vi "Record Measurement.vi"(0 "Linear Density":dbl, 1 "Operator ID":i32, 2 "sMDT Code":string, 4 "Wire Length":dbl, 6 "Tension":dbl, 7 "User List":string[](array[string]), 8 "Uncertainty":dbl, 9 "Frequency":dbl, 10 "Nth measurement":i32, 11 "t < X ?":bool) -> (3 "Measurements":string[][](array[string]))   [LabVIEW 2018]
panel:
  # "Inputs"
  # "Outputs"
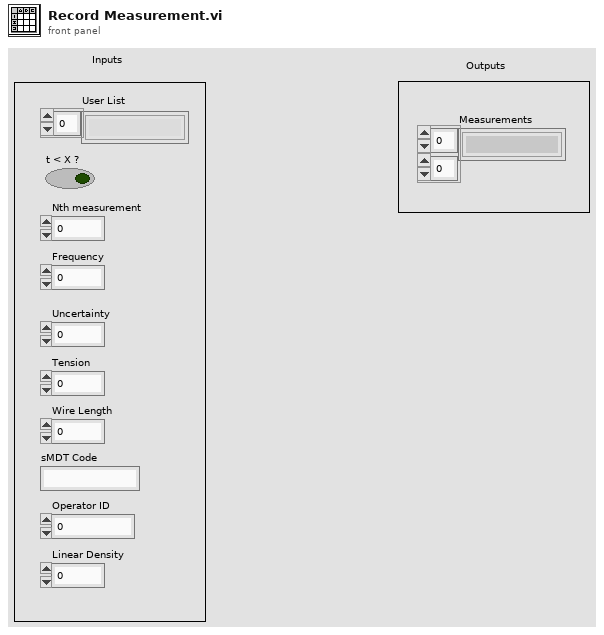
[diagram p1: front panel]
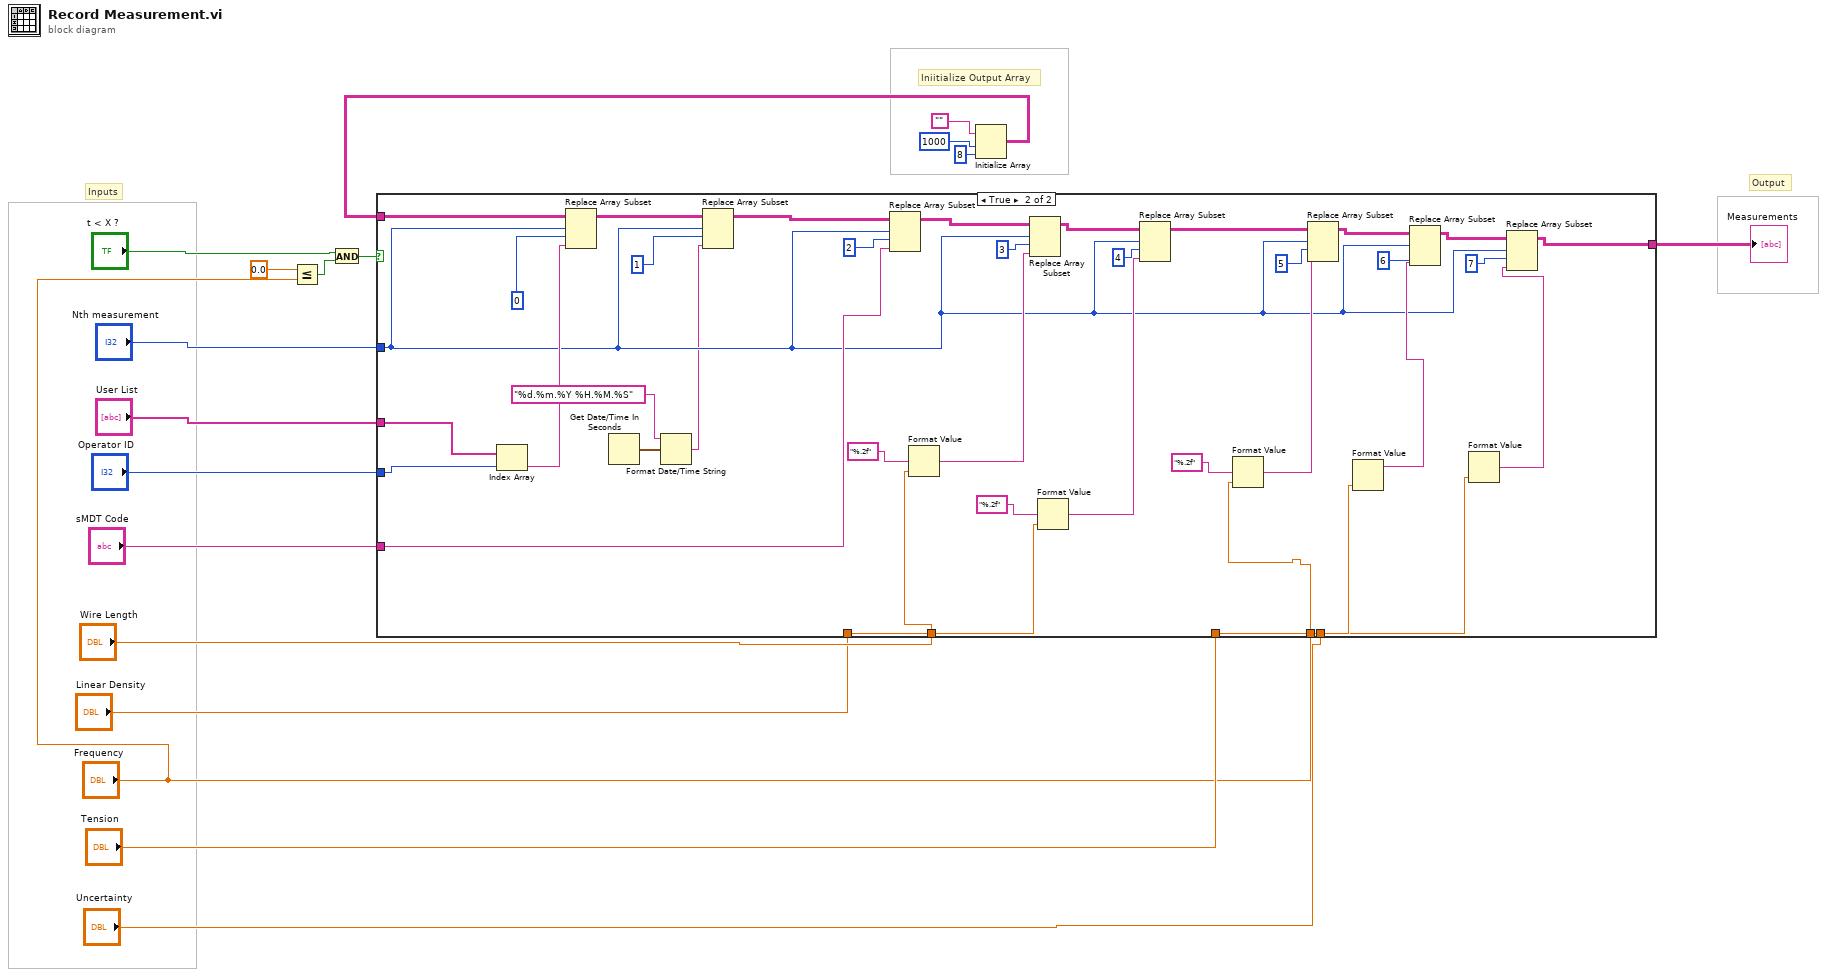
[diagram p0: block diagram]
diagram:
  # "Output"
  # "Inputs"
  # "Iniitialize Output Array"
  n1 = Less Or Equal?(x=0.0, y="Frequency") -> (x <= y?=w5:bool)
  n2 = And(x="t < X ?", y=w5) -> (x .and. y?=w7:bool)
  n3 = Initialize Array("", 1000, 8) -> (w1:string[][])
  n4 = case shown="True" w7 {
    tunnel: w1 -> [w19 w55]
    tunnel: [w19 w31] -> w2
    tunnel: "Nth measurement" -> [_ w23]
    tunnel: "Tension" -> [_ w46]
    tunnel: "Frequency" -> [_ w49]
    tunnel: "User List" -> [_ w51]
    tunnel: "Wire Length" -> [_ w42]
    tunnel: "Linear Density" -> [_ w41]
    tunnel: "sMDT Code" -> [_ w33]
    tunnel: "Operator ID" -> [_ w32]
    tunnel: "Uncertainty" -> [_ w28]
    frame False {
    }
    frame True {
      n5 = Index Array(array=w51, index=w32) -> (element=w50:string)
      n6 = Replace Array Subset(array=w55, new element=w50, index (row)=w23, index (col)=0) -> (w26:string[][])
      n7 = Get Date/Time In Seconds() -> (seconds since 1Jan1904=w22:timestamp)
      n8 = Format Date/Time String(time format string (%c)="%d.%m.%Y %H.%M.%S", seconds (now)=w22) -> (date/time string=w21:string)  [unwired: 1 in]
      n9 = Replace Array Subset(array=w26, new element=w21, index (row)=w23, index (col)=1) -> (w25:string[][])
      n10 = Replace Array Subset(array=w25, new element=w33, index (row)=w23, index (col)=2) -> (w40:string[][])
      n11 = Format Value(format string="%.2f", value (0)=w42) -> (output string=w35:string)  [unwired: 1 in]
      n12 = Replace Array Subset(array=w40, new element=w35, index (row)=w23, index (col)=3) -> (w39:string[][])
      n13 = Format Value(format string="%.2f", value (0)=w41) -> (output string=w34:string)  [unwired: 1 in]
      n14 = Replace Array Subset(array=w39, new element=w34, index (row)=w23, index (col)=4) -> (w38:string[][])
      n15 = Format Value(format string="%.2f", value (0)=w49) -> (output string=w48:string)  [unwired: 1 in]
      n16 = Replace Array Subset(array=w38, new element=w48, index (row)=w23, index (col)=5) -> (w54:string[][])
      n17 = Format Value(value (0)=w46) -> (output string=w47:string)  [unwired: 2 in]
      n18 = Replace Array Subset(array=w54, new element=w47, index (row)=w23, index (col)=6) -> (w30:string[][])
      n19 = Format Value(value (0)=w28) -> (output string=w27:string)  [unwired: 2 in]
      n20 = Replace Array Subset(array=w30, new element=w27, index (row)=w23, index (col)=7) -> (w31:string[][])
    }
  }
  "Measurements" <- w2
